vi "Retrieve Local Repository.vi"(8 "error in":errorcluster, 11 "Artifactory":refnum<class "Artifactory.lvclass">) -> (0 "error out":errorcluster, 1 "found":bool, 2 "Local Repository":path, 3 "Artifactory out":refnum<class "Artifactory.lvclass">)   [LabVIEW 2021, in "Artifactory.lvclass"]
uses:
  Artifactory.lvclass
  Actions -- enum.ctl
  ce154d5c-452a-41ea-87b9-4093452ee6f0.vi
  <vilib>/JDP Science/JSONtext/Find Item.vi
  <vilib>/JDP Science/JSONtext/String Subset.vi
  <vilib>/Utility/error.llb/Error Cluster From Error Code.vi
  <vilib>/JDP Science/JSONtext/Parsing/Parse Full Path or Item Name.vi
  <vilib>/JDP Science/JSONtext/Next JSON Value.vi
  <vilib>/JDP Science/JSONtext/support/Error Cluster From Code.vi
  <vilib>/JDP Science/JSONtext/Offset/Find Item Locations by Path.vi
  <vilib>/JDP Science/JSONtext/JSON text to Variant.vi
  <vilib>/ErrorRing/Error Ring.xnode
  <vilib>/JDP Science/JSONtext/LVClass Serializer/JSONtext LVClass Serializer.lvclass
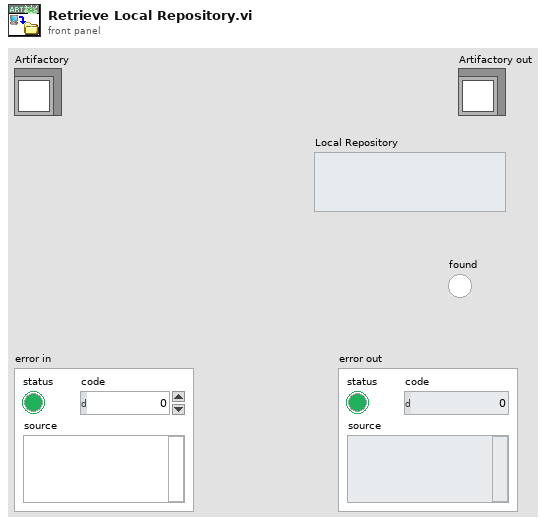
[diagram p1: front panel]
types:
  T1 = typedef "Artifactory.lvclass/Actions -- enum.ctl" = enum16{"Idle", "Custom Event", "Connecting to Artifactory", "Verifying Permissions", "Listing local repository", "Listing remote repository", "Computing changes", "Uploading file", "Downloading file"}
  T2 = enum16{"open", "replace", "create", "open or create", "replace or create", "replace or create with confirmation"}
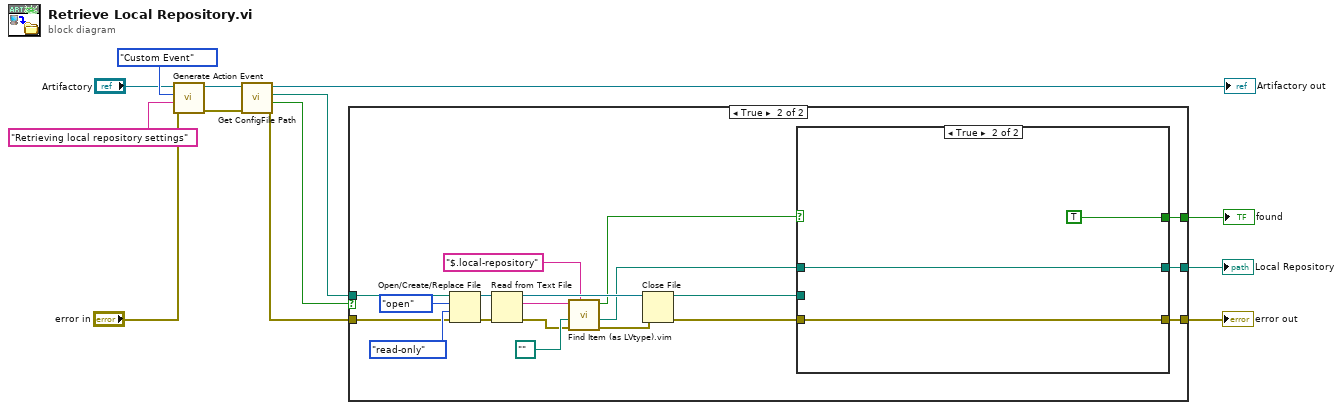
[diagram p0: block diagram]
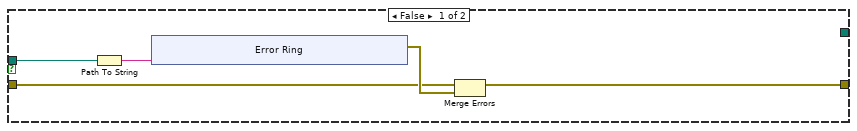
[diagram p2: hidden frame]
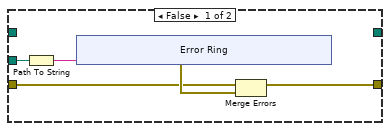
[diagram p3: hidden frame]
diagram:
  n1 = call-dynamic "Generate Action Event.vi"("error in (no error)"="error in", "Description"="Retrieving local repository settings" ("$Path or Item Name"), "Action"=Actions_--_enum."Custom Event", "Artifactory in"="Artifactory") -> ("error out"=w1:errorcluster, "Artifactory out"=w4:refnum<class "Artifactory.lvclass">)  [unwired: 6 in]
  n2 = call-dynamic "Get ConfigFile Path.vi"("error in (no error)"=w1, "Artifactory in"=w4) -> ("error out"=w10:errorcluster, "found"=w11:bool, "Config File"=w12:path, "Artifactory out"=→"Artifactory out":refnum<class "Artifactory.lvclass">)  [unwired: 6 in]
  n3 = case shown="True" w11 {
    tunnel: [w17 w37] -> w9
    tunnel: [_ w36] -> w8
    tunnel: w10 -> [w16 w39]
    tunnel: w12 -> [w15 w38]
    tunnel: [_ w35] -> w7
    frame False {
      n4 = Path To String(path=w15) -> (string=w14:string)
      n5 = xnode "Error Ring"("parameter 0"=w14) -> ("error out"=w18:errorcluster)
      n6 = Merge Errors(w16, w18) -> (w17:errorcluster)
    }
    frame True {
      n7 = Open/Create/Replace File(file path (use dialog)=w38, error in=w39, operation (0:open)=T2."open", access (0:read/write)=enum16{"read/write", "read-only", "write-only"}."read-only") -> (refnum out=w44:refnum<file>, error out=w42:errorcluster)  [unwired: 2 in, 1 out]
      n8 = Read from Text File(file (use dialog)=w44, error in=w42) -> (refnum out=w41:refnum<file>, text=w32:string, error out=w28:errorcluster)  [unwired: 2 in, 1 out]
      n9 = call "Find Item (as LVtype).vim"("$Path or Item Name"="$.local-repository", "error in (no error)"=w28, "Data Type and Default Value"=path "" ("Local Repository"), "JSON"=w32) -> ("error out"=w27:errorcluster, "Data"=w26:path, "Found"=w29:bool)  [unwired: 4 in, 1 out]
      n10 = Close File(refnum=w41, error in=w27) -> (path=w33:path, error out=w34:errorcluster)
      n11 = case shown="True" w29 {
        tunnel: w34 -> [w48 w59]
        tunnel: [w47 w59] -> w37
        tunnel: [_ w57] -> w36
        tunnel: [_ TRUE] -> w35
        tunnel: w26 -> [_ w57]
        tunnel: w33 -> [w46 _]
        frame False {
          n12 = Path To String(path=w46) -> (string=w45:string)
          n13 = xnode "Error Ring"("parameter 0"=w45) -> ("error out"=w49:errorcluster)
          n14 = Merge Errors(w48, w49) -> (w47:errorcluster)
        }
        frame True {
        }
      }
    }
  }
  "error out" <- w9
  "Local Repository" <- w8
  "found" <- w7
